vi "Find Module Main VI.vi"(11 "Module Path":path) -> (3 "Main.vi Path":path)   [LabVIEW 2016, in "PantherLAB_Scripting.lvlib"]
uses:
  PantherLAB_Scripting.lvlib
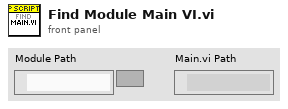
[diagram p1: front panel]
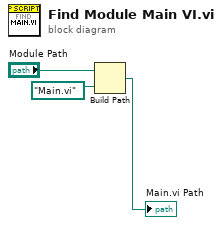
[diagram p0: block diagram]
diagram:
  n1 = Build Path(base path="Module Path", name or relative path=path "Main.vi") -> (appended path=→"Main.vi Path":path)
